vi "Convert Annulus to Sector Parameter.vi"(10 "Annulus":T2={"Center X"=929, "Center Y"=663, "Inner Radius"=200, "Outer Radius"=405, "Start Angle"=90.0, "End Angle"=180.0} {"End Angle" format="%.2f"; "Start Angle" format="%.2f"; "Center X" scale=0.0..1024.0}, 11 "NumWingSectors":u8) -> (3 "Sector Parameter":T1)   [LabVIEW 2013]
uses:
  FPGA/Sector/Accumulate/Sector Parameter Cluster.ctl
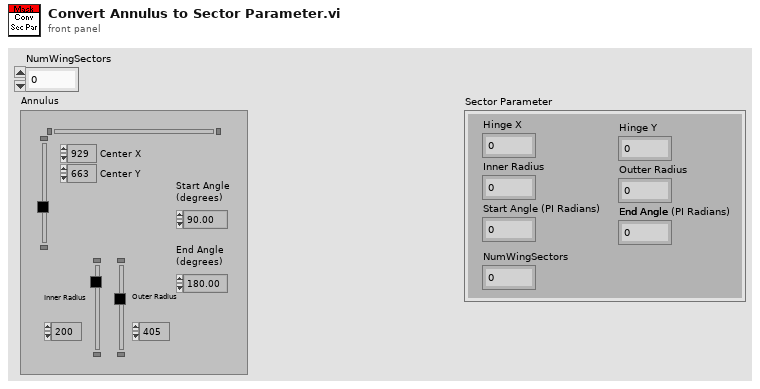
[diagram p1: front panel]
types:
  T1 = typedef "Sector Parameter Cluster.ctl" = cluster{"Start Angle":fxp<+/-,17,2>, "End Angle":fxp<+/-,17,2>, "Inner Radius":u16, "Outter Radius":u16, "Hinge X":u16, "Hinge Y":u16, "NumWingSectors":u8}
  T2 = typedef "IMAQ Circle" = cluster{"Center X":i32, "Center Y":i32, "Inner Radius":i32, "Outer Radius":i32, "Start Angle":dbl, "End Angle":dbl}
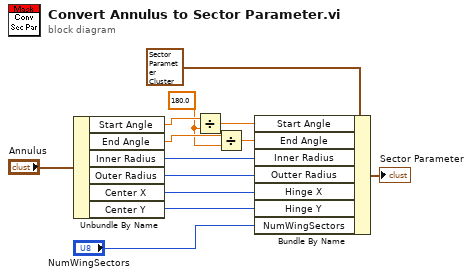
[diagram p0: block diagram]
diagram:
  w8 = 180.0 ("y")
  n1 = Unbundle By Name("Annulus") -> ("Start Angle"=w11:dbl, "End Angle"=w9:dbl, "Inner Radius"=w6:i32, "Outer Radius"=w5:i32, "Center X"=w4:i32, "Center Y"=w3:i32)
  n2 = Divide(x=w11, y=w8) -> (x/y=w10:dbl)
  n3 = Divide(x=w9, y=w8) -> (x/y=w7:dbl)
  n4 = Bundle By Name(cluster=T1 {"Start Angle"=0.65740966796875, "End Angle"=0.99468994140625, "Inner Radius"=309, "Outter Radius"=405, "Hinge X"=464, "Hinge Y"=534, "NumWingSectors"=16} ("Left Sector Parameters"), "Start Angle"=w10, "End Angle"=w7, "Inner Radius"=w6, "Outter Radius"=w5, "Hinge X"=w4, "Hinge Y"=w3, "NumWingSectors"="NumWingSectors") -> (→"Sector Parameter":T1)
